vi "Postflight Position.vi"(0 "error in (no error)":errorcluster) -> (1 "function return":i32, 2 "error out":errorcluster)   [LabVIEW 2014, in "ThorPMT.lvlib"]
doc: "long PostflightPosition();"
uses:
  ThorPMT.lvlib
  ThorPMT.dll
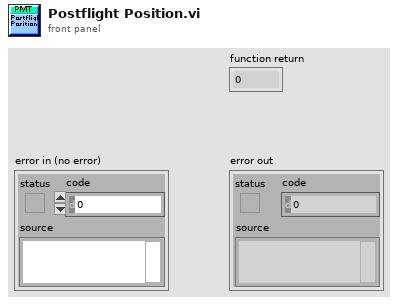
[diagram p1: front panel]
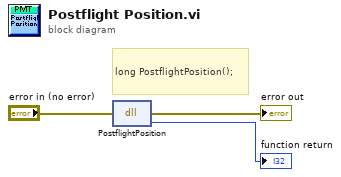
[diagram p0: block diagram]
diagram:
  # "long PostflightPosition();"
  n1 = dll-call lib="C:/TIS_CalebVS2012/TIS_Development/Hardware/SDKs/PMT_SDK/LabVIEW/inc/ThorPMT.*" fn="PostflightPosition"(error in="error in (no error)") -> (error out=→"error out":errorcluster, →"function return":i32)  [unwired: 2 in, 1 out]
